vi "ExTestXCamSameGraph.vi"() -> ()   [LabVIEW 2010]
uses:
  GlbCamHndls.vi
panel:
  in  "Camera Number":u32=1 min=1 max=20 step=1
  out "Camera 1":sgl[](graph)
  in  "stop":bool
  in  "Exposure":dbl=0.5 format="%.2f"
  out "error out":errorcluster
  in  "error in (no error)":errorcluster
  # "ExTestXCamSameGraph:\nThis example runs one  cameras in focus mode.\nSets it up for center strip and displays as graph.\nRemember to setup  cameras in the pvcam.ini\nfile.  For testing multiple camera systems"
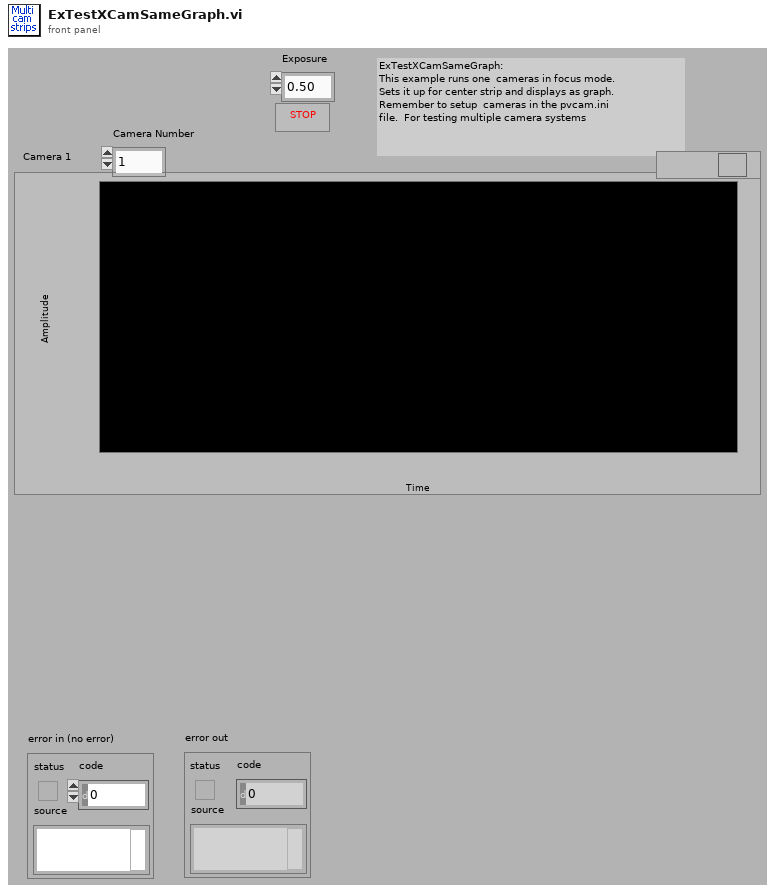
[diagram p1: front panel]
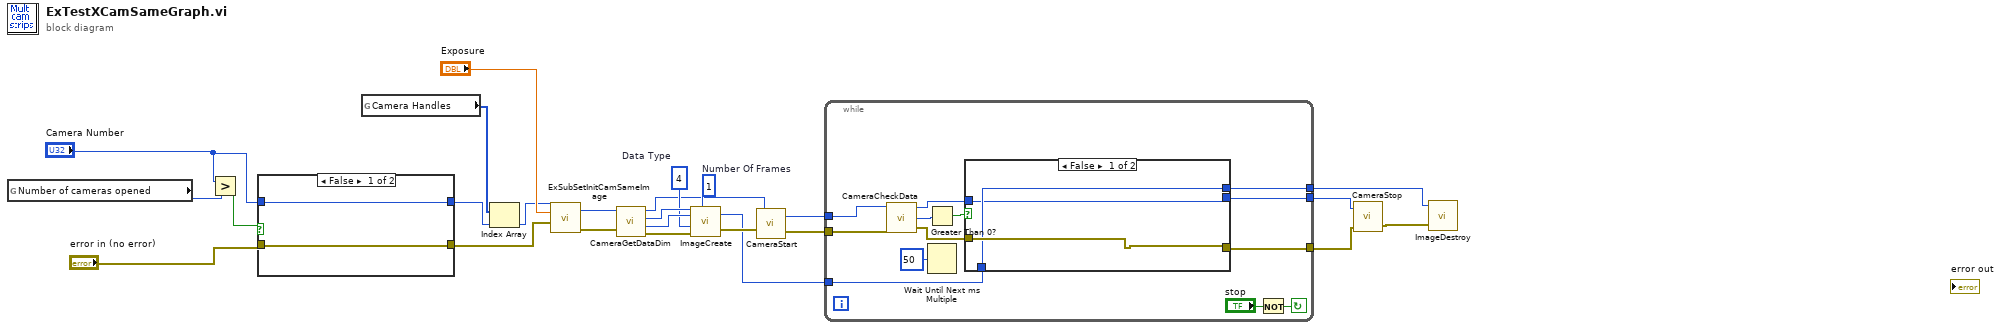
[diagram p0: block diagram]
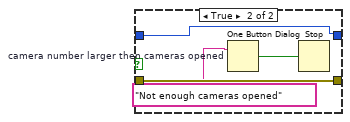
[diagram p2: hidden frame]
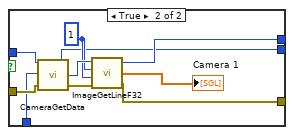
[diagram p3: hidden frame]
diagram:
  w16 = u32 1  # Number Of Frames
  w13 = u32 4  # Data Type
  n1 = global read "GlbCamHndls.vi" "Number of cameras opened"() -> (w22:u32)
  n2 = Greater?(x="Camera Number", y=w22) -> (0:w24:bool)
  n3 = case shown="False" w24 {
    tunnel: "error in (no error)" -> [w27 w31]
    tunnel: [w27 w31] -> w20
    tunnel: "Camera Number" -> [w26 w30]
    tunnel: [w26 w30] -> w18
    frame False {
    }
    frame True {
      n4 = One Button Dialog "camera number larger then cameras opened"(message="Not enough cameras opened") -> (true=w29:bool)  [unwired: 1 in]
      n5 = Stop(stop? (T)=w29) -> ()
    }
  }
  n6 = global read "GlbCamHndls.vi" "Camera Handles"() -> (w12:u32[])
  n7 = Index Array(array=w12, index=w18) -> (element=w21:u32)
  n8 = call "ExSubSetInitCamSameImage.vi"("error in (no error)"=w20, "Exposure"="Exposure", "Camera Handle"=w21) -> ("error out"=w11:errorcluster, "Camera Handle 2"=w10:u32)
  n9 = call <userlib>:"CameraGetDataDim.vi"("Camera Handle"=w10, "error in"=w11) -> ("Camera Handle"=w3:u32, "Xdim"=w15:u32, "Ydim"=w14:u32, "error out"=w17:errorcluster)
  n10 = call <userlib>:"ImageCreate.vi"("X dimension"=w15, "Y dimension"=w14, "Data Type"=w13, "error in"=w17, "Number Of Frames"=w16) -> ("Image Handle"=w2:u32, "error out"=w9:errorcluster)
  n11 = call <userlib>:"CameraStart.vi"("error in"=w9, "Camera Handle"=w3) -> ("error out"=w7:errorcluster, "Camera Handle"=w8:u32)
  n12 = while {
    tunnel: w8 -> [w37]
    tunnel: w7 -> [w36]
    tunnel: [w35] -> w6
    tunnel: [w34] -> w4
    tunnel: w2 -> [w33]
    tunnel: [w32] -> w1
    stop <- w43 continue-if-true
    n13 = call <userlib>:"CameraCheckData.vi"("Camera Handle"=w37, "error in"=w36) -> ("Camera Handle"=w39:u32, "Number Of Frames Available"=w41:i32, "error out"=w38:errorcluster)
    n14 = Greater Than 0?(x=w41) -> (x > 0?=w40:bool)
    n15 = Wait Until Next ms Multiple(millisecond multiple=u32 50) -> ()  [unwired: 1 out]
    n16 = case shown="False" w40 {
      tunnel: [w47 w54] -> w35
      tunnel: w39 -> [w45 w53]
      tunnel: w38 -> [w47 w52]
      tunnel: [w46 w50] -> w34
      tunnel: w33 -> [w46 w49]
      tunnel: [w45 w48] -> w32
      frame False {
      }
      frame True {
        w55 = 1
        n17 = call <userlib>:"CameraGetData.vi"("error in"=w52, "Data Handle"=w49, "Camera Handle"=w53) -> ("error out"=w57:errorcluster, "Data Handle"=w56:u32, "Camera Handle"=w48:u32)
        n18 = call <userlib>:"ImageGetLineF32.vi"("error in"=w57, "Z Position"=w55, "Y Position"=w55, "Data Handle"=w56) -> ("error out"=w54:errorcluster, "Array F32"=→"Camera 1":sgl[], "Data Handle"=w50:u32)
      }
    }
    n19 = Not(x="stop") -> (.not. x?=w43:bool)
  }
  n20 = call <userlib>:"CameraStop.vi"("error in"=w6, "Camera Handle"=w1) -> ("error out"=w5:errorcluster)  [unwired: 1 out]
  n21 = call <userlib>:"ImageDestroy.vi"("error in"=w5, "Data handle"=w4) -> ()  [unwired: 1 out]
